vi "TriggerEvent.vi"(6 "Imgs":picture[](array[picture]), 7 "Step Len":dbl, 8 "error in":errorcluster, 9 "Pic Ref":refnum<vi>, 10 "Ctrl Ref":u32, 11 "Command":T1) -> (0 "error out":errorcluster)   [LabVIEW 2012, in "Spinner.xctl"]
uses:
  Spinner.xctl
  Command.ctl
  EventData.ctl
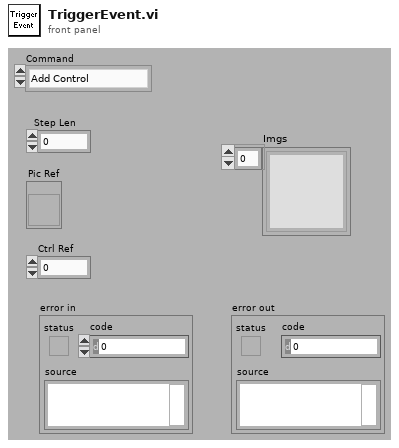
[diagram p1: front panel]
types:
  T1 = typedef "Spinner.xctl/Command.ctl" = enum16{"Add Control", "Remove Control", "Update Imgs", "Update Speed", "Refresh"}
  T2 = typedef "Spinner.xctl/EventData.ctl" = cluster{"Step Len":dbl, "Pic Ref":refnum<vi>, "Ctrl Ref":u32, "Imgs":picture[], "Command":T1}
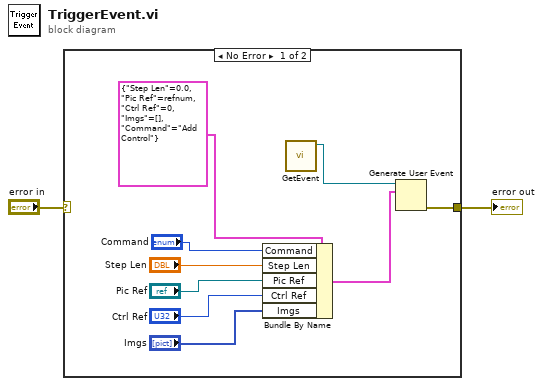
[diagram p0: block diagram]
diagram:
  n1 = case shown="No Error" "error in" {
    selector: "error in" -> [_ w12]
    tunnel: [w7 w12] -> w2
    frame No Error {
      n2 = Bundle By Name(cluster=T2 {"Step Len"=0.0, "Pic Ref"=refnum, "Ctrl Ref"=0, "Imgs"=[], "Command"=enum."Add Control"} ("Spinner event datatype"), "Command"="Command", "Step Len"="Step Len", "Pic Ref"="Pic Ref", "Ctrl Ref"="Ctrl Ref", "Imgs"="Imgs") -> (w3:T2)
      n3 = call "GetEvent.vi"() -> ("Event"=w4:refnum<user-event>)  [unwired: 10 in, 1 out]
      n4 = Generate User Event(user event=w4, event data cluster=w3) -> (error out=w7:errorcluster)  [unwired: 1 in, 1 out]
    }
    frame Error {
    }
  }
  "error out" <- w2
